vi "OnDataChange.vi"(0 "DataListener in":refnum<class "DataListener.lvclass">, 1 "DataExchange":T1, 3 "error in (no error)":errorcluster) -> (7 "DataListener out":refnum<class "DataListener.lvclass">, 10 "error out":errorcluster)   [LabVIEW 2020, in "DataListener.lvclass"]
uses:
  DataListener.lvclass
  Model/Hardware Abstraction Layer/Component/Device/Device/DataExchange.ctl
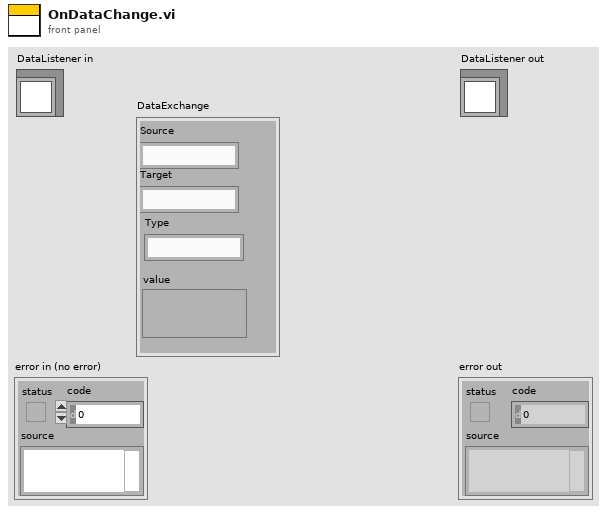
[diagram p1: front panel]
types:
  T1 = typedef "DataListener.lvclass/DataExchange.ctl" = cluster{"Source":string, "Target":string, "Type":string, "value":variant}
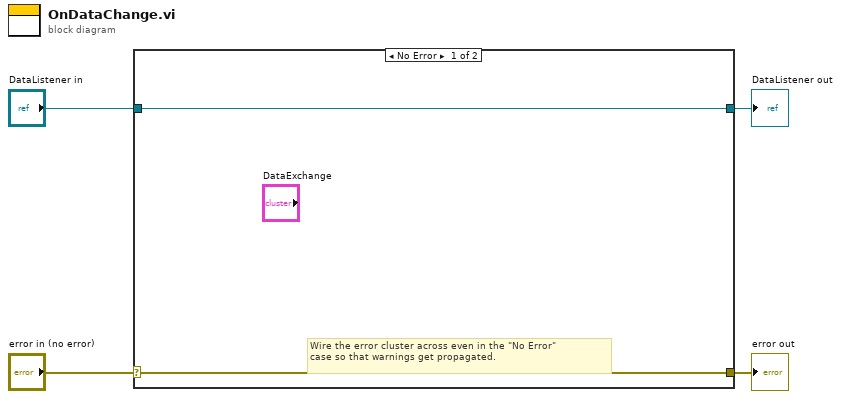
[diagram p0: block diagram]
diagram:
  n1 = case shown="No Error" "error in (no error)" {
    selector: "error in (no error)" -> [w5 w8]
    tunnel: [w5 w8] -> w3
    tunnel: [w6 w7] -> w1
    tunnel: "DataListener in" -> [w6 w7]
    frame No Error {
      # "Wire the error cluster across even in the \"No Error\"\ncase so that warnings get propagated."
    }
    frame Error {
    }
  }
  "error out" <- w3
  "DataListener out" <- w1
